vi "超标留样状态参数解析.vi"(0 "输入字符串":string, 1 "超标留样":T2={"当前瓶号："=0.0, "平行样："=0.0, "留样瓶数："=0.0, "每瓶次数："=0.0, "每次留样："=0.0, "时间间隔："=0.0, "COD联机："=2, "氨氮联机："=2, "4mA浓度："=0.0, "20mA浓度："=0.0, "超标浓度："=0.0, "4mA浓度："=0.0, "20mA浓度:"=0.0, "超标浓度："=0.0} {"COD联机：" items=["继电器"=1, "模拟输入"=2, "串口连接"=3]; "氨氮联机：" items=["继电器"=1, "模拟输入"=2, "串口连接"=3]}, 2 "外控留样":T1, 5 "解析/转指令":enum16{"解析", "转指令"}(ring), 9 "模式选择":enum16{"外控留样", "超标留样"}(ring), 11 "error in (no error)":errorcluster caption="错误输入（无错误）") -> (3 "输出字符串":string, 15 "error out":errorcluster caption="错误输出")   [LabVIEW 2016, in "德润DR803F超标留样.lvlib"]
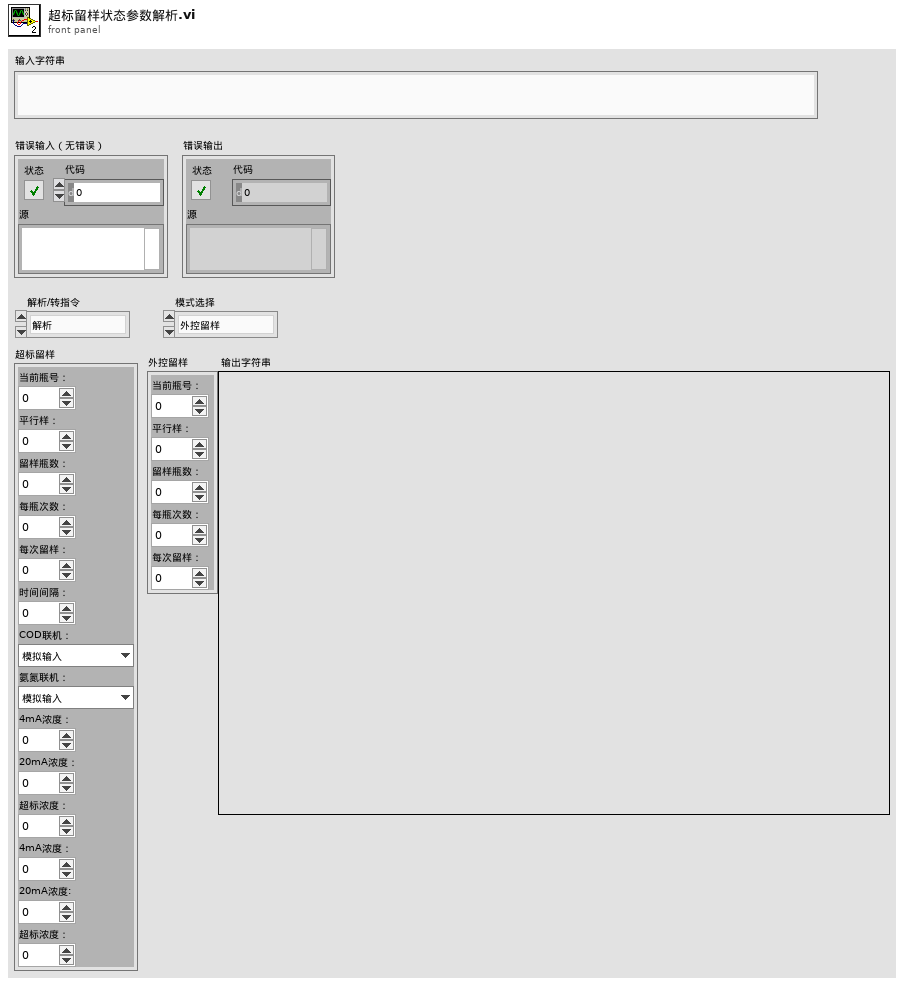
[diagram p1: front panel]
types:
  T1 = cluster{"当前瓶号：":dbl, "平行样：":dbl, "留样瓶数：":dbl, "每瓶次数：":dbl, "每次留样：":dbl}
  T2 = cluster{"当前瓶号：":dbl, "平行样：":dbl, "留样瓶数：":dbl, "每瓶次数：":dbl, "每次留样：":dbl, "时间间隔：":dbl, "COD联机：":u16, "氨氮联机：":u16, "4mA浓度：":dbl, "20mA浓度：":dbl, "超标浓度：":dbl, "4mA浓度：":dbl, "20mA浓度:":dbl, "超标浓度：":dbl}
  T3 = cluster{"采样模式":u16, "当前瓶号：":dbl, "平行样：":dbl, "留样瓶数：":dbl, "每瓶次数：":dbl, "每次留样：":dbl, "时间间隔：":dbl, "COD联机：":u16, "4mA浓度：":dbl, "20mA浓度：":dbl, "超标浓度：":dbl, "当前浓度：":dbl, "氨氮联机：":u16, "4mA浓度：":dbl, "20mA浓度:":dbl, "超标浓度：":dbl, "当前浓度：":dbl}
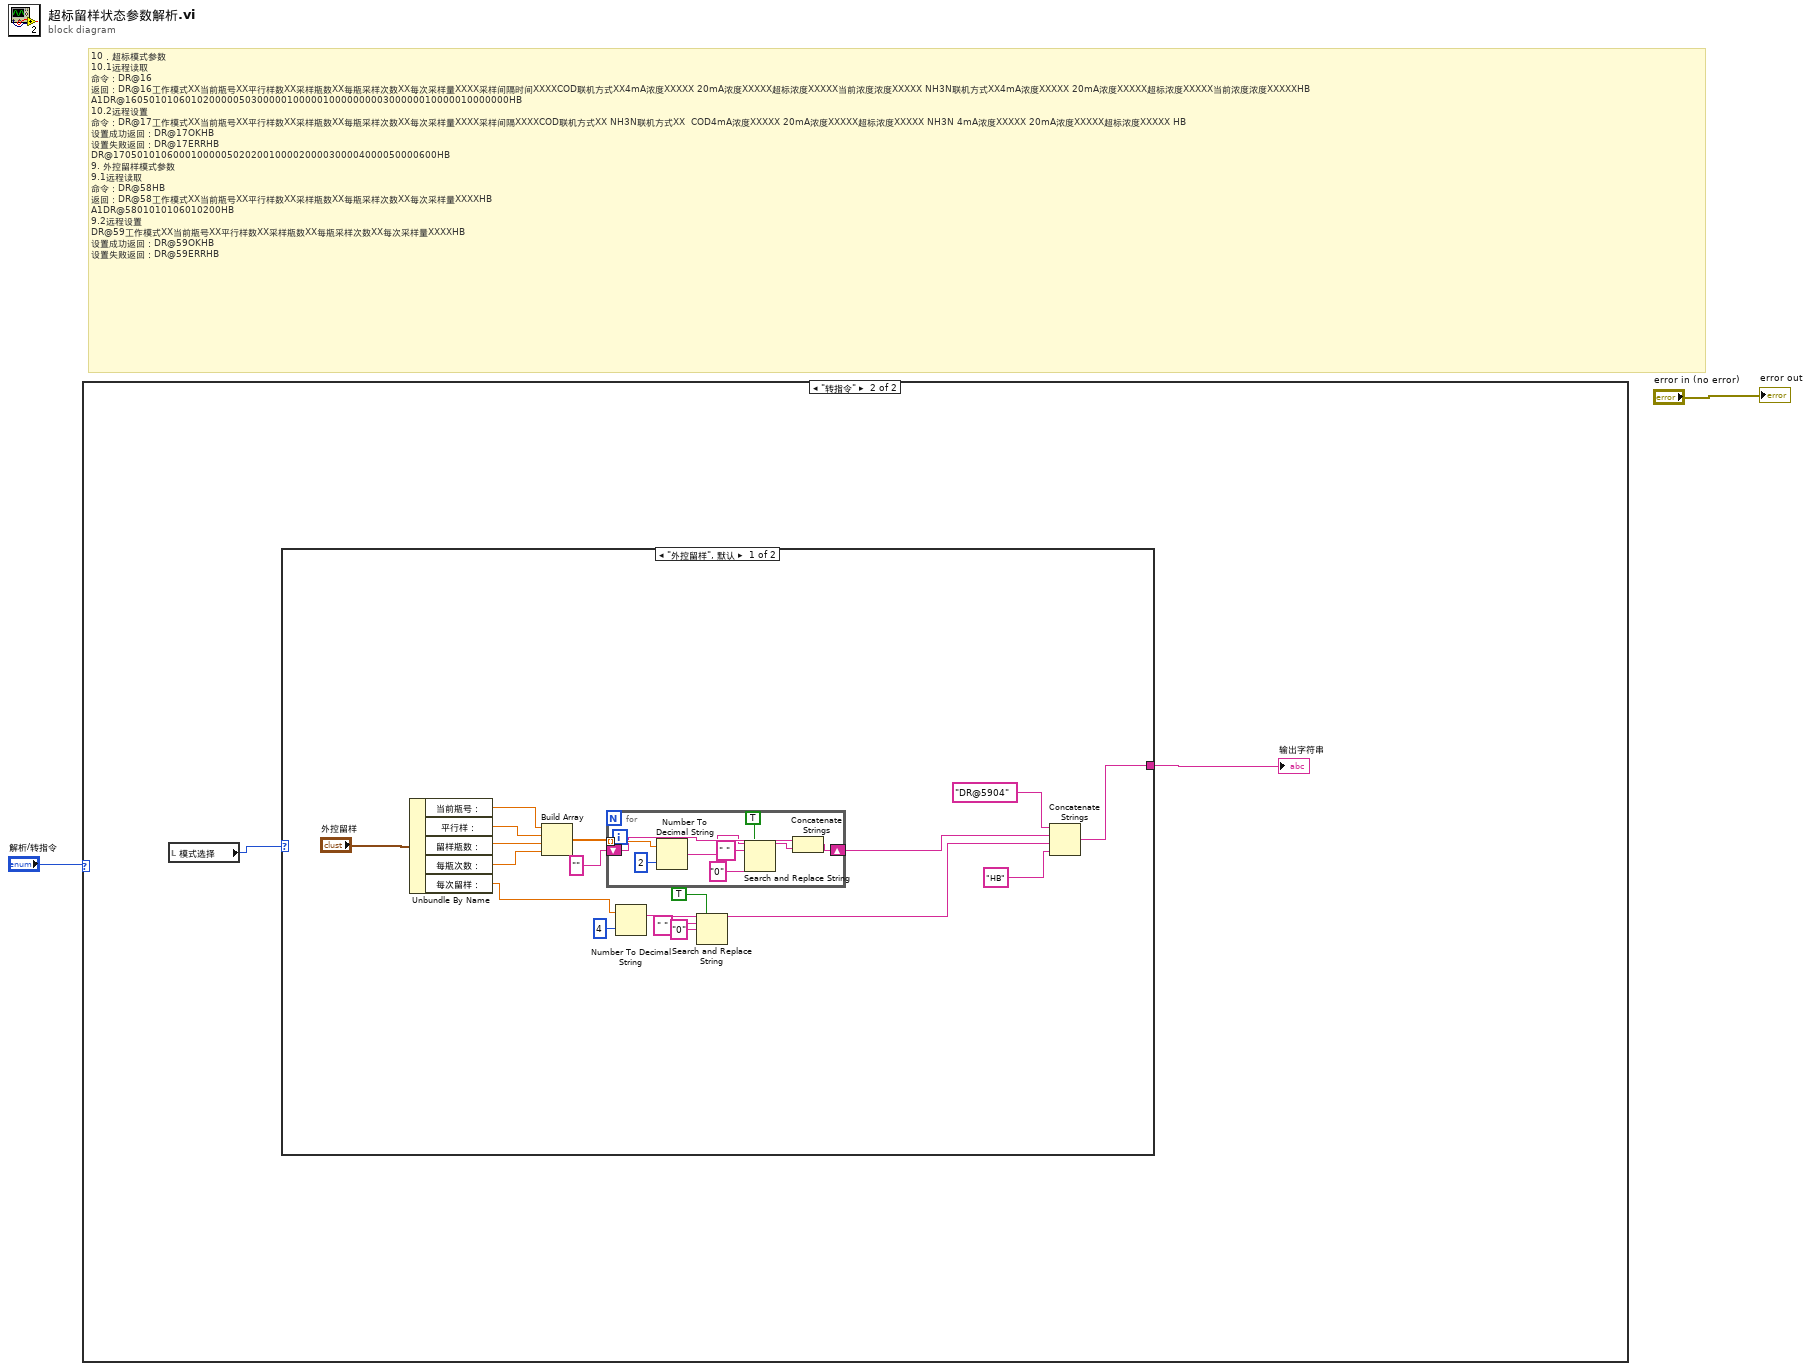
[diagram p0: block diagram]
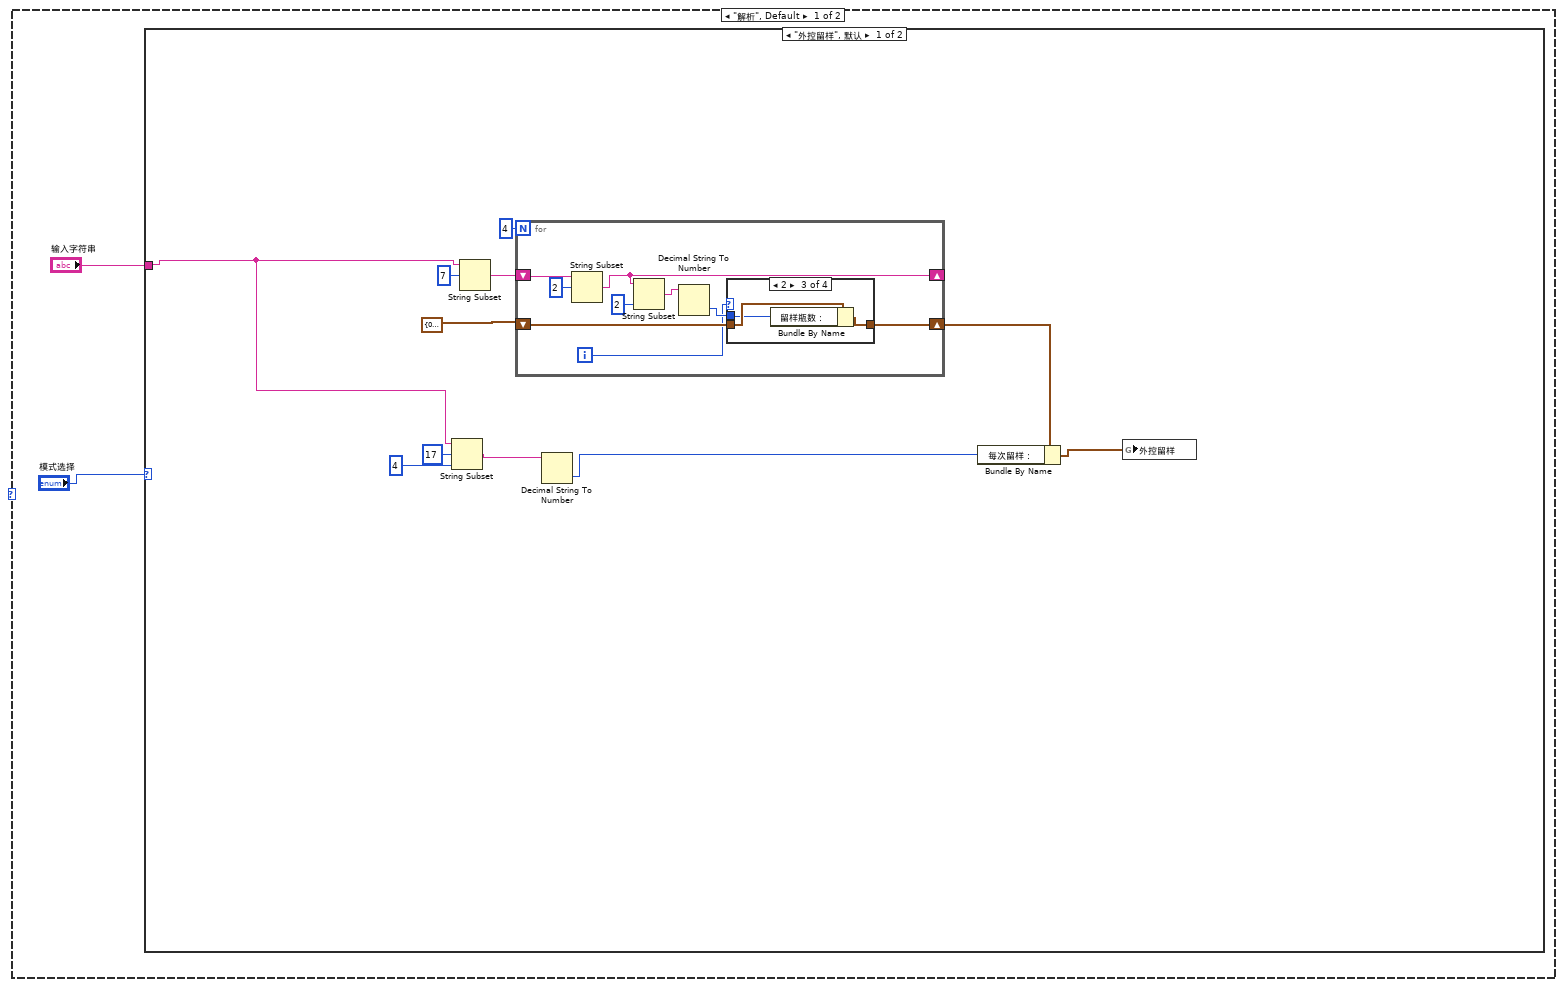
[diagram p2: hidden frame]
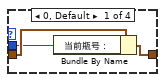
[diagram p3: hidden frame]
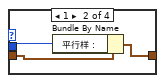
[diagram p4: hidden frame]
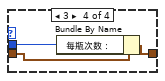
[diagram p5: hidden frame]
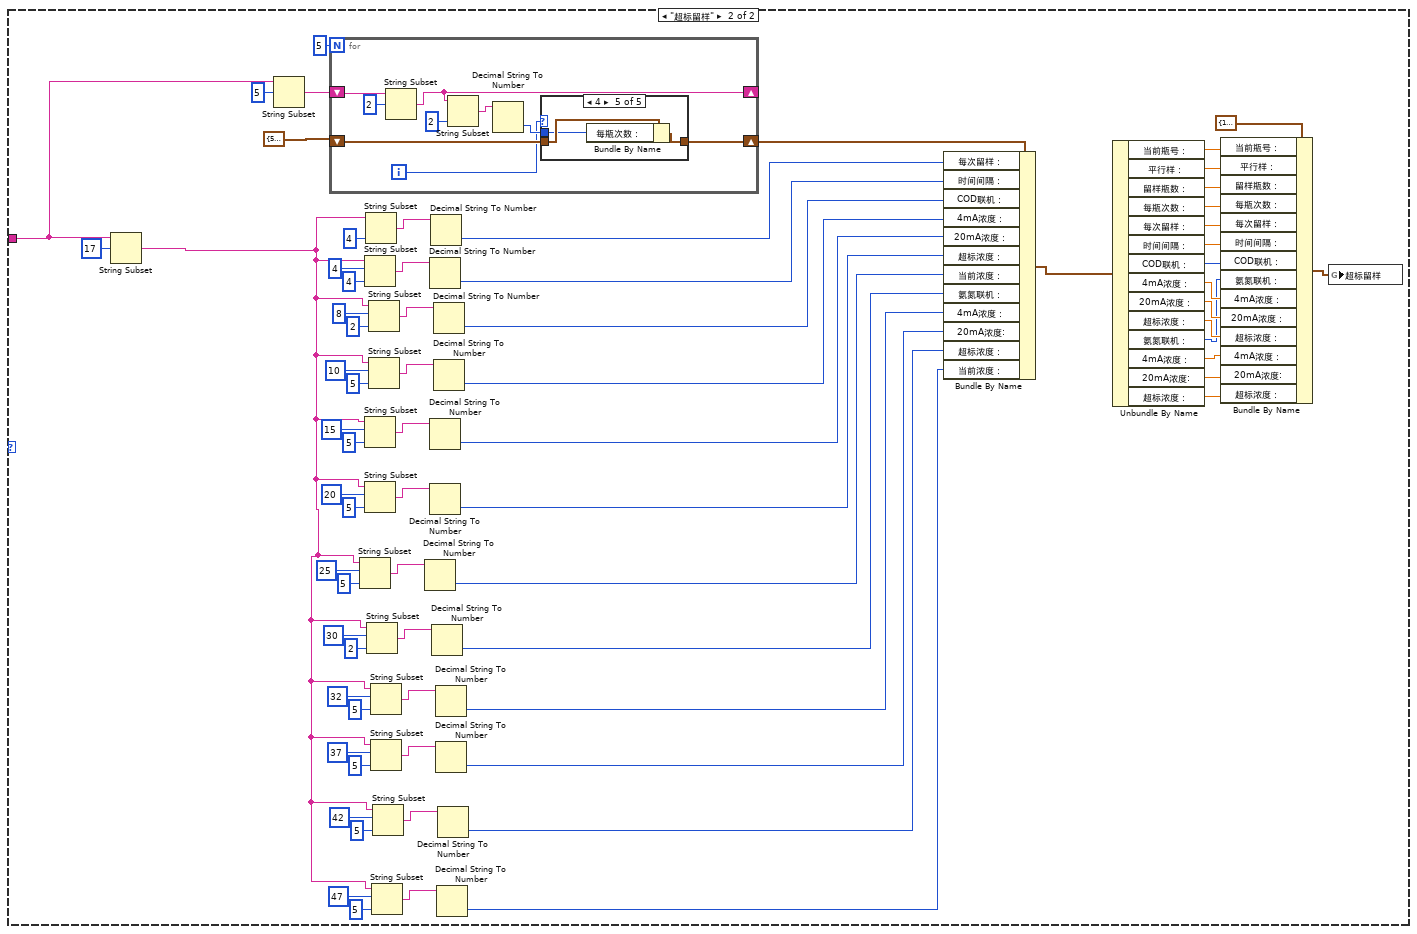
[diagram p6: hidden frame]
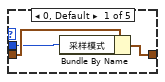
[diagram p7: hidden frame]
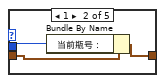
[diagram p8: hidden frame]
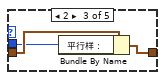
[diagram p9: hidden frame]
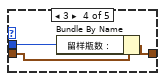
[diagram p10: hidden frame]
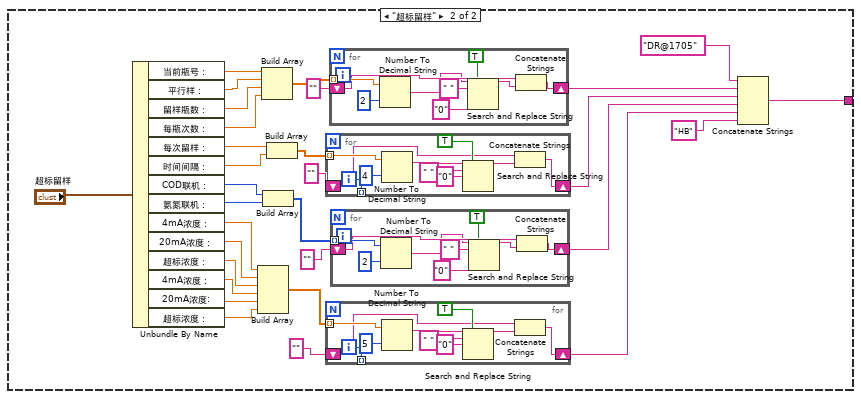
[diagram p11: hidden frame]
diagram:
  # "10．超标模式参数\n10.1远程读取\n命令：DR@16\n返回：DR@16工作模式XX当前瓶号XX平行样数XX采样瓶数XX每瓶采样次数XX每次采样量XXXX采样间隔时间XXXXCOD联机方式XX4mA浓度XXXXX 20mA浓度XXXXX超标浓度XXXXX当前浓度浓度XXXXX NH3N联机方式XX4mA浓度XXXXX 20mA浓度XXXXX超标浓度XXXXX当前浓度浓度XXXXXHB\nA1DR@1605010106010200000503000001000001000000000300000010000010000000HB\n10.2远程设置\n命令：DR@17工作模式XX当前瓶号XX平行样数XX采样瓶数XX每瓶采样次数XX每次采样量XXXX采样间隔XXXXCOD联机方式XX NH3N联机方式XX  COD4mA浓度XXXXX 20mA浓度XXXXX超标浓度XXXXX NH3N 4mA浓度XXXXX 20mA浓度XXXXX超标浓度XXXXX HB\n设置成功返回：DR@17OKHB\n设置失败返回：DR@17ERRHB\nDR@170501010600010000050202001000020000300004000050000600HB\n9. 外控留样模式参数\n9.1远程读取\n命令：DR@58HB\n返回：DR@58工作模式XX当前瓶号XX平行样数XX采样瓶数XX每瓶采样次数XX每次采样量XXXXHB\nA1DR@5801010106010200HB\n9.2远程设置\nDR@59工作模式XX当前瓶号XX平行样数XX采样瓶数XX每瓶采样次数XX每次采样量XXXXHB\n设置成功返回：DR@59OKHB\n设置失败返回：DR@59ERRHB"
  n1 = case shown="\"转指令\"" "解析/转指令" {
    frame "解析", Default {
      n2 = case shown="\"外控留样\", 默认" "模式选择" {
        tunnel: "输入字符串" -> [w10 w86]
        frame "外控留样", Default {
          n3 = String Subset(string=w10, offset (0)=17 ("偏移量(0)"), length (rest)=4 ("长度（剩余）")) -> (substring=w8:string)
          n4 = String Subset(string=w10, offset (0)=7 ("偏移量(0)")) -> (substring=w13:string)  [unwired: 1 in]
          n5 = for {
            N: 4 -> [_]
            shift-right: [w22] -> _
            shift-left: w13 -> [w24]
            shift-right: [w17] -> w7
            shift-left: T1 {"当前瓶号："=0.0, "平行样："=0.0, "留样瓶数："=0.0, "每瓶次数："=0.0, "每次留样："=0.0} ("外控留样") -> [w19]
            i -> [w16]
            n6 = String Subset(string=w24, offset (0)=2 ("偏移量(0)")) -> (substring=w22:string)  [unwired: 1 in]
            n7 = String Subset(string=w22, length (rest)=2 ("长度（剩余）")) -> (substring=w20:string)  [unwired: 1 in]
            n8 = Decimal String To Number(string=w20) -> (number=w18:i32)  [unwired: 2 in, 1 out]
            n9 = case shown="2" w16 {
              tunnel: w19 -> [w27 w29 w33 w36]
              tunnel: w18 -> [w26 w28 w32 w34]
              tunnel: [w25 w30 w31 w35] -> w17
              frame 0, Default {
                n10 = Bundle By Name(cluster=w27, "当前瓶号："=w26) -> (w25:T1)
              }
              frame 1 {
                n11 = Bundle By Name(cluster=w29, "平行样："=w28) -> (w30:T1)
              }
              frame 2 {
                n12 = Bundle By Name(cluster=w33, "留样瓶数："=w32) -> (w31:T1)
              }
              frame 3 {
                n13 = Bundle By Name(cluster=w36, "每瓶次数："=w34) -> (w35:T1)
              }
            }
          }
          n14 = Decimal String To Number(string=w8) -> (number=w6:i32)  [unwired: 2 in, 1 out]
          n15 = Bundle By Name(cluster=w7, "每次留样："=w6) -> (w5:T1)
          n16 = global write "超标留样全局.vi" "外控留样"(w5) -> ()
        }
        frame "超标留样" {
          n17 = String Subset(string=w86, offset (0)=17 ("偏移量(0)")) -> (substring=w57:string)  [unwired: 1 in]
          n18 = String Subset(string=w86, offset (0)=5 ("偏移量(0)")) -> (substring=w105:string)  [unwired: 1 in]
          n19 = for {
            N: 5 -> [_]
            shift-right: [w115] -> _
            shift-left: w105 -> [w117]
            shift-right: [w110] -> w104
            shift-left: T3 {"采样模式"=5, "当前瓶号："=1.0, "平行样："=1.0, "留样瓶数："=6.0, "每瓶次数："=1.0, "每次留样："=200.0, "时间间隔："=5.0, "COD联机："=3, "4mA浓度："=0.0, "20mA浓度："=0.0, "超标浓度："=0.0, "当前浓度："=0.0, "氨氮联机："=2, "4mA浓度："=0.0, "20mA浓度:"=0.0, "超标浓度："=0.0, "当前浓度："=0.0} ("超标留样") -> [w112]
            i -> [w109]
            n20 = String Subset(string=w117, offset (0)=2 ("偏移量(0)")) -> (substring=w115:string)  [unwired: 1 in]
            n21 = String Subset(string=w115, length (rest)=2 ("长度（剩余）")) -> (substring=w113:string)  [unwired: 1 in]
            n22 = Decimal String To Number(string=w113) -> (number=w111:i32)  [unwired: 2 in, 1 out]
            n23 = case shown="4" w109 {
              tunnel: w112 -> [w120 w122 w126 w129 w132]
              tunnel: w111 -> [w119 w121 w125 w127 w130]
              tunnel: [w118 w123 w124 w128 w131] -> w110
              frame 0, Default {
                n24 = Bundle By Name(cluster=w120, "采样模式"=w119) -> (w118:T3)
              }
              frame 1 {
                n25 = Bundle By Name(cluster=w122, "当前瓶号："=w121) -> (w123:T3)
              }
              frame 2 {
                n26 = Bundle By Name(cluster=w126, "平行样："=w125) -> (w124:T3)
              }
              frame 3 {
                n27 = Bundle By Name(cluster=w129, "留样瓶数："=w127) -> (w128:T3)
              }
              frame 4 {
                n28 = Bundle By Name(cluster=w132, "每瓶次数："=w130) -> (w131:T3)
              }
            }
          }
          n29 = String Subset(string=w57, offset (0)=25 ("偏移量(0)"), length (rest)=5 ("长度（剩余）")) -> (substring=w78:string)
          n30 = String Subset(string=w57, offset (0)=4 ("偏移量(0)"), length (rest)=4 ("长度（剩余）")) -> (substring=w101:string)
          n31 = String Subset(string=w57, offset (0)=15 ("偏移量(0)"), length (rest)=5 ("长度（剩余）")) -> (substring=w90:string)
          n32 = String Subset(string=w57, offset (0)=20 ("偏移量(0)"), length (rest)=5 ("长度（剩余）")) -> (substring=w87:string)
          n33 = String Subset(string=w57, length (rest)=4 ("长度（剩余）")) -> (substring=w102:string)  [unwired: 1 in]
          n34 = String Subset(string=w57, offset (0)=30 ("偏移量(0)"), length (rest)=2 ("长度（剩余）")) -> (substring=w72:string)
          n35 = String Subset(string=w57, offset (0)=8 ("偏移量(0)"), length (rest)=2 ("长度（剩余）")) -> (substring=w96:string)
          n36 = String Subset(string=w57, offset (0)=10 ("偏移量(0)"), length (rest)=5 ("长度（剩余）")) -> (substring=w95:string)
          n37 = String Subset(string=w57, offset (0)=32 ("偏移量(0)"), length (rest)=5 ("长度（剩余）")) -> (substring=w70:string)
          n38 = String Subset(string=w57, offset (0)=37 ("偏移量(0)"), length (rest)=5 ("长度（剩余）")) -> (substring=w67:string)
          n39 = String Subset(string=w57, offset (0)=47 ("偏移量(0)"), length (rest)=5 ("长度（剩余）")) -> (substring=w58:string)
          n40 = String Subset(string=w57, offset (0)=42 ("偏移量(0)"), length (rest)=5 ("长度（剩余）")) -> (substring=w66:string)
          n41 = Decimal String To Number(string=w78) -> (number=w75:i32)  [unwired: 2 in, 1 out]
          n42 = Decimal String To Number(string=w101) -> (number=w84:i32)  [unwired: 2 in, 1 out]
          n43 = Decimal String To Number(string=w90) -> (number=w80:i32)  [unwired: 2 in, 1 out]
          n44 = Decimal String To Number(string=w87) -> (number=w79:i32)  [unwired: 2 in, 1 out]
          n45 = Decimal String To Number(string=w102) -> (number=w85:i32)  [unwired: 2 in, 1 out]
          n46 = Decimal String To Number(string=w72) -> (number=w71:i32)  [unwired: 2 in, 1 out]
          n47 = Decimal String To Number(string=w96) -> (number=w83:i32)  [unwired: 2 in, 1 out]
          n48 = Decimal String To Number(string=w95) -> (number=w81:i32)  [unwired: 2 in, 1 out]
          n49 = Decimal String To Number(string=w70) -> (number=w63:i32)  [unwired: 2 in, 1 out]
          n50 = Decimal String To Number(string=w67) -> (number=w62:i32)  [unwired: 2 in, 1 out]
          n51 = Decimal String To Number(string=w58) -> (number=w56:i32)  [unwired: 2 in, 1 out]
          n52 = Decimal String To Number(string=w66) -> (number=w61:i32)  [unwired: 2 in, 1 out]
          n53 = Bundle By Name(cluster=w104, "每次留样："=w85, "时间间隔："=w84, "COD联机："=w83, "4mA浓度："=w81, "20mA浓度："=w80, "超标浓度："=w79, "当前浓度："=w75, "氨氮联机："=w71, "4mA浓度："=w63, "20mA浓度:"=w62, "超标浓度："=w61, "当前浓度："=w56) -> (w52:T3)
          n54 = Unbundle By Name(w52) -> ("当前瓶号："=w51:dbl, "平行样："=w50:dbl, "留样瓶数："=w49:dbl, "每瓶次数："=w48:dbl, "每次留样："=w47:dbl, "时间间隔："=w46:dbl, "COD联机："=w45:u16, "4mA浓度："=w44:dbl, "20mA浓度："=w43:dbl, "超标浓度："=w42:dbl, "氨氮联机："=w41:u16, "4mA浓度："=w40:dbl, "20mA浓度:"=w39:dbl, "超标浓度："=w38:dbl)
          n55 = Bundle By Name(cluster=T2 {"当前瓶号："=1.0, "平行样："=0.0, "留样瓶数："=6.0, "每瓶次数："=0.0, "每次留样："=100.0, "时间间隔："=5.0, "COD联机："=2, "氨氮联机："=2, "4mA浓度："=0.0, "20mA浓度："=0.0, "超标浓度："=0.0, "4mA浓度："=0.0, "20mA浓度:"=0.0, "超标浓度："=0.0} ("超标留样"), "当前瓶号："=w51, "平行样："=w50, "留样瓶数："=w49, "每瓶次数："=w48, "每次留样："=w47, "时间间隔："=w46, "COD联机："=w45, "氨氮联机："=w41, "4mA浓度："=w44, "20mA浓度："=w43, "超标浓度："=w42, "4mA浓度："=w40, "20mA浓度:"=w39, "超标浓度："=w38) -> (w37:T2)
          n56 = global write "超标留样全局.vi" "超标留样"(w37) -> ()
        }
      }
    }
    frame "转指令" {
      n57 = local read "模式选择"() -> (w133:enum16{"外控留样", "超标留样"})
      n58 = case shown="\"外控留样\", 默认" w133 {
        tunnel: [w144 w162] -> w134
        frame "外控留样", Default {
          n59 = Unbundle By Name("外控留样") -> ("当前瓶号："=w151:dbl, "平行样："=w150:dbl, "留样瓶数："=w149:dbl, "每瓶次数："=w148:dbl, "每次留样："=w137:dbl)
          n60 = Build Array(w151, w150, w149, w148) -> (w147:dbl[])
          n61 = for {
            tunnel: w147 -> [w160] mode=indexing
            shift-right: [w153] -> w143
            shift-left: "" -> [w159]
            n62 = Number To Decimal String(number=w160, width (-)=i16 2 ("宽度(-)")) -> (decimal integer string=w154:string)
            n63 = Search and Replace String(replace all?=TRUE ("替换全部？(F)"), input string=w154, search string=" " ("搜索字符串"), replace string="0" ("替换字符串(\"\")")) -> (result string=w155:string)  [unwired: 4 in, 3 out]
            n64 = Concatenate Strings(w159, w155) -> (w153:string)
          }
          n65 = Number To Decimal String(number=w137, width (-)=i16 4 ("宽度(-)")) -> (decimal integer string=w140:string)
          n66 = Search and Replace String(replace all?=TRUE ("替换全部？(F)"), input string=w140, search string=" " ("搜索字符串"), replace string="0" ("替换字符串(\"\")")) -> (result string=w136:string)  [unwired: 4 in, 3 out]
          n67 = Concatenate Strings("DR@5904" ("字符串"), w143, w136, "HB" ("字符串")) -> (w144:string)
        }
        frame "超标留样" {
          n68 = Unbundle By Name("超标留样") -> ("当前瓶号："=w189:dbl, "平行样："=w190:dbl, "留样瓶数："=w191:dbl, "每瓶次数："=w185:dbl, "每次留样："=w184:dbl, "时间间隔："=w183:dbl, "COD联机："=w180:u16, "氨氮联机："=w179:u16, "4mA浓度："=w176:dbl, "20mA浓度："=w175:dbl, "超标浓度："=w174:dbl, "4mA浓度："=w173:dbl, "20mA浓度:"=w172:dbl, "超标浓度："=w171:dbl)
          n69 = Build Array(w176, w175, w174, w173, w172, w171) -> (w169:dbl[])
          n70 = Build Array(w189, w190, w191, w185) -> (w188:dbl[])
          n71 = Build Array(w180, w179) -> (w178:u16[])
          n72 = Build Array(w184, w183) -> (w182:dbl[])
          n73 = for {
            tunnel: w182 -> [w220] mode=indexing
            shift-right: [w212] -> w166
            shift-left: "" -> [w213]
            tunnel: [w211] -> _ mode=indexing
            i -> [w211]
            n74 = Number To Decimal String(number=w220, width (-)=i16 4 ("宽度(-)")) -> (decimal integer string=w217:string)
            n75 = Search and Replace String(replace all?=TRUE ("替换全部？(F)"), input string=w217, search string=" " ("搜索字符串"), replace string="0" ("替换字符串(\"\")")) -> (result string=w214:string)  [unwired: 4 in, 3 out]
            n76 = Concatenate Strings(w213, w214) -> (w212:string)
          }
          n77 = for {
            tunnel: w169 -> [w201] mode=indexing
            shift-right: [w193] -> w164
            shift-left: "" -> [w194]
            tunnel: [w192] -> _ mode=indexing
            i -> [w192]
            n78 = Number To Decimal String(number=w201, width (-)=i16 5 ("宽度(-)")) -> (decimal integer string=w198:string)
            n79 = Search and Replace String(replace all?=TRUE ("替换全部？(F)"), input string=w198, search string=" " ("搜索字符串"), replace string="0" ("替换字符串(\"\")")) -> (result string=w195:string)  [unwired: 4 in, 3 out]
            n80 = Concatenate Strings(w194, w195) -> (w193:string)
          }
          n81 = for {
            tunnel: w188 -> [w228] mode=indexing
            shift-right: [w221] -> w167
            shift-left: "" -> [w227]
            n82 = Number To Decimal String(number=w228, width (-)=i16 2 ("宽度(-)")) -> (decimal integer string=w222:string)
            n83 = Search and Replace String(replace all?=TRUE ("替换全部？(F)"), input string=w222, search string=" " ("搜索字符串"), replace string="0" ("替换字符串(\"\")")) -> (result string=w223:string)  [unwired: 4 in, 3 out]
            n84 = Concatenate Strings(w227, w223) -> (w221:string)
          }
          n85 = for {
            tunnel: w178 -> [w209] mode=indexing
            shift-right: [w202] -> w165
            shift-left: "" -> [w208]
            n86 = Number To Decimal String(number=w209, width (-)=i16 2 ("宽度(-)")) -> (decimal integer string=w203:string)
            n87 = Search and Replace String(replace all?=TRUE ("替换全部？(F)"), input string=w203, search string=" " ("搜索字符串"), replace string="0" ("替换字符串(\"\")")) -> (result string=w204:string)  [unwired: 4 in, 3 out]
            n88 = Concatenate Strings(w208, w204) -> (w202:string)
          }
          n89 = Concatenate Strings("DR@1705" ("字符串"), w167, w166, w165, w164, "HB" ("字符串")) -> (w162:string)
        }
      }
      "输出字符串" <- w134
    }
  }
  "error out" <- "error in (no error)"
